vi "SaveAsTiff.vi"(7 "Data In":u16[][](array[numeric]), 8 "Header In":T1={"header info"={"Header"="", "Head length"=0}, "A/D info"={"# rf points per line"=0, "# lines per scan"=0, "sample rate MHz"=0, "# A/D bits"=0, "# bytes per A/D"=0, "TGC Flag"=0, "A/D Type"=""}, "Tranducer Info"={"bandwidth"=0.0, "center freq"=0.0, "start freq"=0.0, "ID"=0}, "Scan Info"={"delay"=0.0, "pivot distance"=0.0, "sector scan angle"=0.0, "operator"="", "Scan Mode"="", "location"=""}, "Time/Date Info"={"date"="", "time"=""}, "RF Info"={"RF file name"="", "RF file att"="", "RF cal file name"="", "RF cal file att"=""}, "Patient Info"={"ID"="", "extended ID"="", "age"=0, "sex"="", "previously\nscanned"="", "PSA"=0.0, "LOS"=1, "Ethnicty 2"=3, "Race"=3}, "Tissue Type"={"organ"=0, "disease type"=0, "disease location"=0, "IQ_pts"=0, "RcvBuffer"=0, "RcvFrame"=0, "IQBuff"=0, "IQFrame"=0, "IQPage"=0}, "Votage scaling"={"Digitizer (dB)"=0.0, "Gain (dB)"=0.0, "Atten (dB)"=0.0}, "Comment"="", "Misc Info"={"avg num"=0, "c speed"=0, "Div By or SF zones"=0, "XMIT CHS"=0, "RCV CHS"=0, "Xmit angle"=0.0}, "Therapy Parameters"={"Theraputic Freq (MHz)"=0.0, "Time on (s)"=0.0, "Therapy amplitude (mV)"=0.0, "Lines Before"=0, "Lines After"=0}, "Scan Settings"={"Energy (uJ or V)"=0, "Damp (Ohm) or Fc"=0, "HP Filt (KHz)"=0, "LP Filt (MHz)"=0, "Gain (db)"=0, "prf (kHz)"=0.0, "Distance between\nscan lines (um)"=0, "Distance between\nscan planes (um)"=0, "Scan line gap (um)"=0.0, "Scan plane gap (um)"=0.0}, "Compression Parameters"={"F1 (MHz)"=0.0, "F2 (MHz)"=0.0, "% taper"=0.0, "duration"=0.0}, "Patient Info Xtra"={"First Name"="", "Last Name"="", "Notes"=""}, "ROI Box"=[0, 0, 0, 0]} {"Compression Parameters"."% taper" min=50 max=1000 format="%.2f"; "Compression Parameters"."F2 (MHz)" format="%.3f"; "Compression Parameters"."F1 (MHz)" format="%.3f"; "Scan Settings"."prf (kHz)" format="%.2f"; "Therapy Parameters"."Therapy amplitude (mV)" min=50 max=1000 format="%.2f"; "Therapy Parameters"."Time on (s)" format="%.3f"; "Therapy Parameters"."Theraputic Freq (MHz)" format="%.3f"; "Patient Info"."Race" items=["Am Ind or Alaska", "Asian", "Hawaiian, Pac Isl", "Black or Afr Amer", "White", "more than one race", "unknown"]; "Patient Info"."Ethnicty 2" items=["Hispanic", "Non-Hispanic", "unknown"]; "Patient Info"."LOS" items=["1", "2", "3", "4", "5"]; "Patient Info"."PSA" format="%.1f"; "Scan Info"."delay" format="%.2f"; "Scan Info"."pivot distance" format="%.2f"; "Scan Info"."sector scan angle" format="%.2f"; "Tranducer Info"."bandwidth" format="%.2f"; "Tranducer Info"."center freq" format="%.2f"; "Tranducer Info"."start freq" format="%.2f"}, 9 "File Path":path, 10 "Image Name":string="untitled", 11 "pairs":dbl) -> ()   [LabVIEW 2022 SP3]
uses:
  ViewData/-ReadEye/Header.ctl
  <vilib>/Analysis/NI_AALPro.lvlib
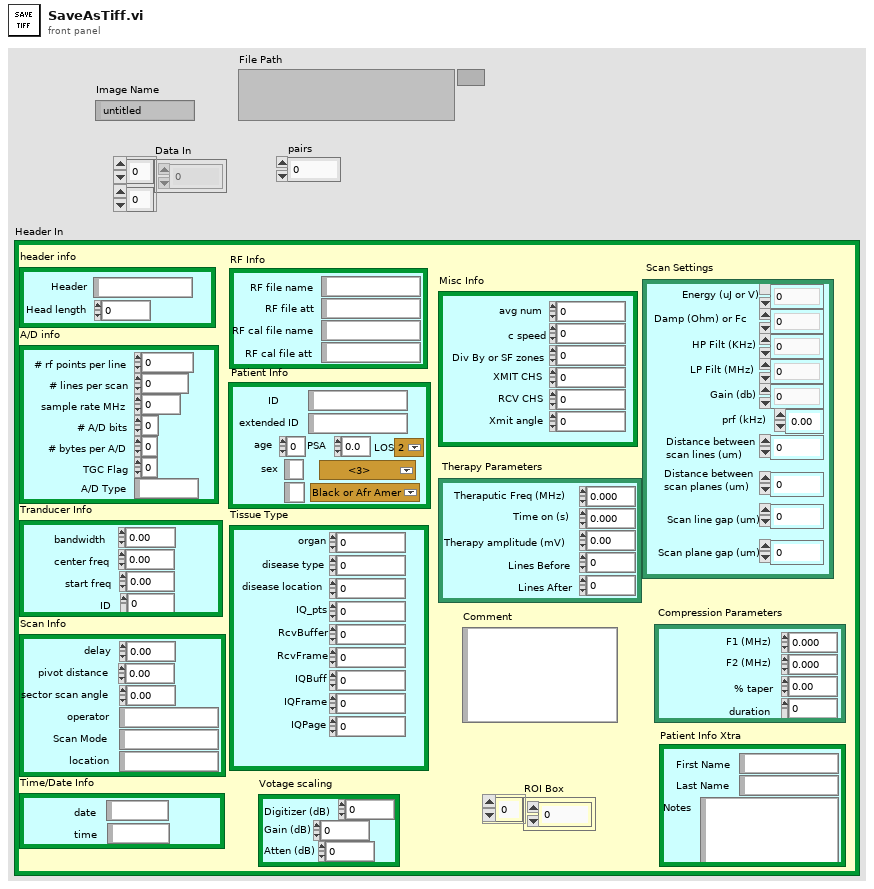
[diagram p1: front panel]
types:
  T1 = typedef "Header.ctl" = cluster{"header info":cluster{"Header":string, "Head length":i16}, "A/D info":cluster{"# rf points per line":u16, "# lines per scan":u16, "sample rate MHz":u16, "# A/D bits":i16, "# bytes per A/D":u16, "TGC Flag":u16, "A/D Type":string}, "Tranducer Info":cluster{"bandwidth":sgl, "center freq":sgl, "start freq":sgl, "ID":i32}, "Scan Info":cluster{"delay":sgl, "pivot distance":sgl, "sector scan angle":sgl, "operator":string, "Scan Mode":string, "location":string}, "Time/Date Info":cluster{"date":string, "time":string}, "RF Info":cluster{"RF file name":string, "RF file att":string, "RF cal file name":string, "RF cal file att":string}, "Patient Info":cluster{"ID":string, "extended ID":string, "age":u16, "sex":string, "previously\nscanned":string, "PSA":sgl, "LOS":u8, "Ethnicty 2":u8, "Race":u8}, "Tissue Type":cluster{"organ":i16, "disease type":i16, "disease location":i16, "IQ_pts":u16, "RcvBuffer":u8, "RcvFrame":u16, "IQBuff":u8, "IQFrame":u16, "IQPage":u8}, "Votage scaling":cluster{"Digitizer (dB)":sgl, "Gain (dB)":sgl, "Atten (dB)":sgl}, "Comment":string, "Misc Info":cluster{"avg num":u16, "c speed":i16, "Div By or SF zones":i16, "XMIT CHS":u8, "RCV CHS":u8, "Xmit angle":sgl}, "Therapy Parameters":cluster{"Theraputic Freq (MHz)":sgl, "Time on (s)":sgl, "Therapy amplitude (mV)":sgl, "Lines Before":u16, "Lines After":u16}, "Scan Settings":cluster{"Energy (uJ or V)":u8, "Damp (Ohm) or Fc":u8, "HP Filt (KHz)":u8, "LP Filt (MHz)":u8, "Gain (db)":u8, "prf (kHz)":sgl, "Distance between\nscan lines (um)":u16, "Distance between\nscan planes (um)":u16, "Scan line gap (um)":sgl, "Scan plane gap (um)":sgl}, "Compression Parameters":cluster{"F1 (MHz)":sgl, "F2 (MHz)":sgl, "% taper":sgl, "duration":sgl}, "Patient Info Xtra":cluster{"First Name":string, "Last Name":string, "Notes":string}, "ROI Box":u16[]}
  T2 = typedef "Image Type" = u32
  T3 = typedef "IMAQ Image.ctl" = refnum<image>
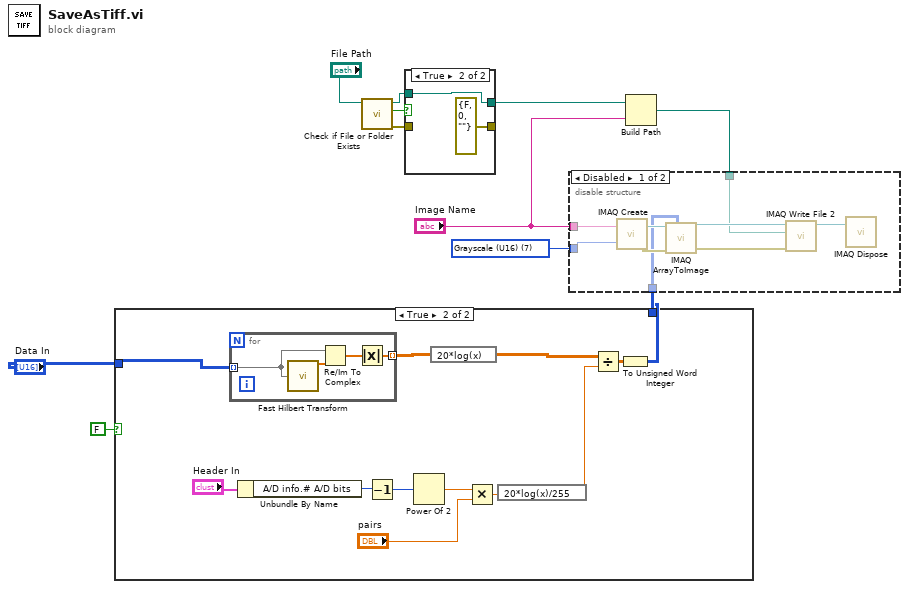
[diagram p0: block diagram]
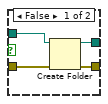
[diagram p4: hidden frame]
diagram:
  w11 = T2 7 items=["Grayscale (U8)", "Grayscale (I16)", "Grayscale (SGL)", "Complex (CSG)", "RGB (U32)", "HSL (U32)", "RGB (U64)", "Grayscale (U16)"] ("Image Type")
  n1 = case shown="True" FALSE {
    tunnel: "Data In" -> [w12 w16]
    tunnel: [w12 w13] -> w1
    frame False {
    }
    frame True {
      n2 = for {
        tunnel: [w26] -> w15 mode=indexing
        tunnel: w16 -> [w25] mode=indexing
        n3 = call <vilib>:"Fast Hilbert Transform.vi"("X"=w25) -> ("Hilbert{X}"=w28:dbl[])  [unwired: 1 out]
        n4 = Re/Im To Complex(1:w28, 2:w25) -> (0:w27:cdb[])
        n5 = Absolute Value(x=w27) -> (abs(x)=w26:dbl[])
      }
      n6 = Unbundle By Name("Header In") -> ("A/D info.# A/D bits"=w22:i16)
      n7 = Decrement(x=w22) -> (x-1=w23:i16)
      n8 = Power Of 2(x=w23) -> (2^x=w21:dbl)
      n9 = expression code="20*log(x)"(w15) -> (w17:dbl[][])
      n10 = Multiply(x=w21, y="pairs") -> (x*y=w19:dbl)
      n11 = expression code="20*log(x)/255"(w19) -> (w18:dbl)
      n12 = Divide(x=w17, y=w18) -> (x/y=w14:dbl[][])
      n13 = To Unsigned Word Integer(number=w14) -> (unsigned 16bit integer=w13:u16[][])
    }
  }
  n14 = call <vilib>:"Check if File or Folder Exists.vi"("path"="File Path") -> ("error out"=w10:errorcluster, "file or folder exists?"=w8:bool, "dup path"=w9:path)  [unwired: 8 in]
  n15 = case shown="True" w8 {
    tunnel: w10 -> [w32 _]
    tunnel: w9 -> [w31 w33]
    tunnel: [w30 errorcluster {"status"=FALSE, "code"=0, "source"=""} ("error out")] -> _
    tunnel: [w29 w33] -> w6
    frame False {
      n16 = Create Folder(path (use dialog)=w31, error in=w32) -> (created path=w29:path, error out=w30:errorcluster)  [unwired: 1 in, 1 out]
    }
    frame True {
    }
  }
  n17 = Build Path(base path=w6, name or relative path="Image Name") -> (appended path=w4:path)
  n18 = disable-structure shown="Disabled" {
    disable-tunnel: w11 -> [w43 _]
    disable-tunnel: "Image Name" -> [w37 _]
    disable-tunnel: w4 -> [w36 _]
    disable-tunnel: w1 -> [w35 _]
    frame Disabled {
      n19 = call "IMAQ Create"("Image Name"=w37, "Image Type"=w43) -> ("New Image"=w40:T3, "error out"=w38:errorcluster)  [unwired: 3 in]
      n20 = call "IMAQ ArrayToImage"("Image Pixels (U16)"=w35, "error in (no error)"=w38, "Image"=w40) -> ("error out"=w39:errorcluster, "Image Out"=w41:T3)  [unwired: 7 in]
      n21 = call-poly "IMAQ Write File 2"("error in (no error)"=w39, "File Path"=w36, "Image"=w41) -> ("Image Out (duplicate)"=w42:T3)  [unwired: 7 in, 1 out]
      n22 = call "IMAQ Dispose"("Image"=w42) -> ()  [unwired: 5 in, 1 out]
    }
    frame Enabled {
    }
  }
